vi "读取数据.vi"(8 "error in (no error)":errorcluster, 11 "基本数据类型.lvclass in":refnum<class "基本数据类型.lvclass">) -> (0 "error out":errorcluster, 2 "数据":dbl, 3 "基本数据类型.lvclass out":refnum<class "基本数据类型.lvclass">)   [LabVIEW 2021, in "基本数据类型.lvclass"]
doc: "本VI是为《我和LabVIEW》一书编写的示例。\n关于本书的介绍请参考网页：\nhttp://ruanqizhen.spaces.live.com/blog/cns!5852D4F797C53FB6!4310.entry"
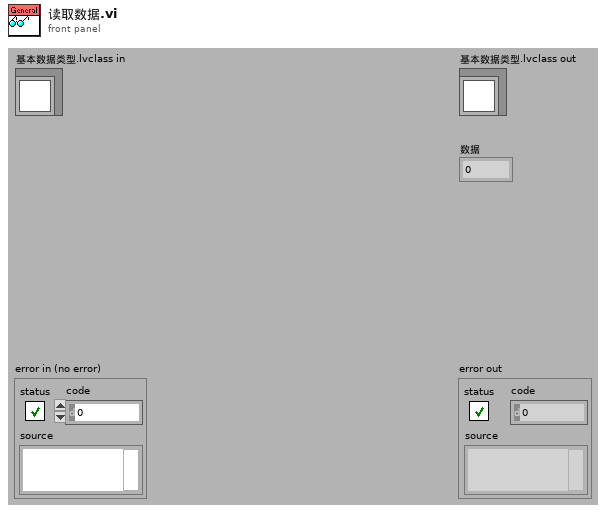
[diagram p1: front panel]
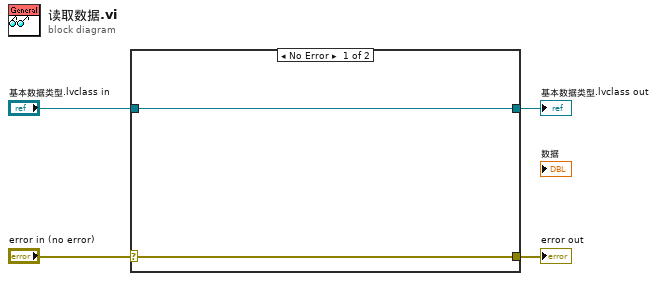
[diagram p0: block diagram]
diagram:
  n1 = case shown="No Error" "error in (no error)" {
    selector: "error in (no error)" -> [w6 w7]
    tunnel: [w6 w7] -> w3
    tunnel: [w5 w8] -> w1
    tunnel: "基本数据类型.lvclass in" -> [w5 w8]
    frame No Error {
    }
    frame Error {
    }
  }
  "error out" <- w3
  "基本数据类型.lvclass out" <- w1
